vi "Get Signature.vi"(6 "offset":i32, 8 "error in (no error)":errorcluster, 11 "bitfile xml in":string) -> (0 "error out":errorcluster, 3 "Bitfile Signature":string, 4 "offset past EndTag":i32)   [LabVIEW 2010, in "FPGA Bitfile Utility.lvlib"]
uses:
  <userlib>/_FPGA Interface Advanced Tools/FPGA Bitfile Utility/FPGA Bitfile Utility.lvlib
  <vilib>/rvi/Utilities/XML/nirviXML_GetValue_String.vi
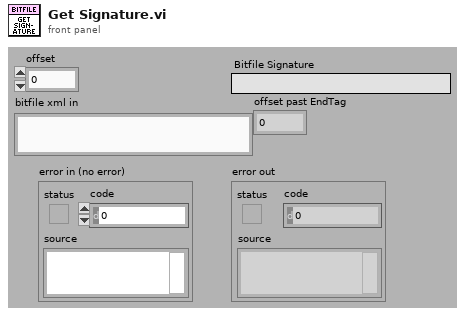
[diagram p1: front panel]
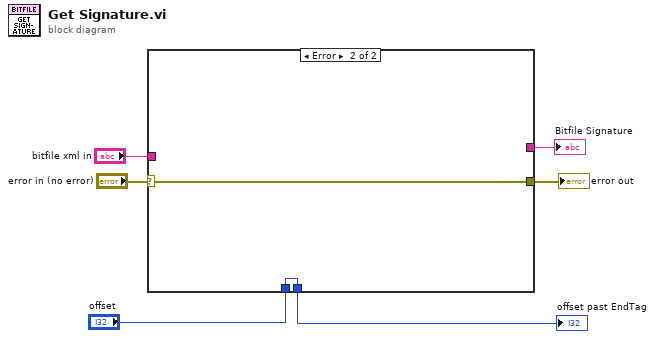
[diagram p0: block diagram]
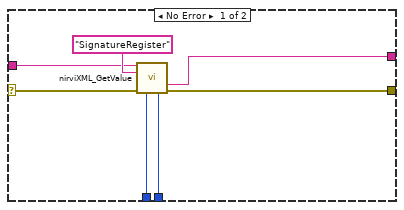
[diagram p2: hidden frame]
diagram:
  n1 = case shown="Error" "error in (no error)" {
    selector: "error in (no error)" -> [w10 w15]
    tunnel: [w12 w15] -> w5
    tunnel: [w11 _] -> w4
    tunnel: "bitfile xml in" -> [w9 _]
    tunnel: "offset" -> [w8 w14]
    tunnel: [w7 w14] -> w1
    frame No Error {
      n2 = call-poly <vilib>:"nirviXML_GetValue.vi"("xml string in"=w9, "tag name in"="SignatureRegister" ("tag"), "error in (no error)"=w10, "offset"=w8) -> ("value"=w11:string, "offset past EndTag"=w7:i32, "error out"=w12:errorcluster)  [unwired: 1 in, 8 out]
    }
    frame Error {
    }
  }
  "error out" <- w5
  "Bitfile Signature" <- w4
  "offset past EndTag" <- w1
